vi "ImportExperiment.vi"(8 "error in (no error)":errorcluster, 10 "Tuple":T1={"mouse_id"=1217.0, "exp_date"="", "operator"="Manolis", "mass"=0.0, "anesthesia"="fentanyl", "directory"="", "dyes"="OGB", "exp_notes"="", "setup"="2P1", "archive"="", "process"="yes"}, 11 "Database in":refnum<class "Database.lvclass">) -> (0 "error out":errorcluster, 3 "Database out":refnum<class "Database.lvclass">)   [LabVIEW 2014, in "Database.lvclass"]
uses:
  Database.lvclass
  Database.lvclass/Database.ctl
  <vilib>/addons/database/NI_Database_API.lvlib
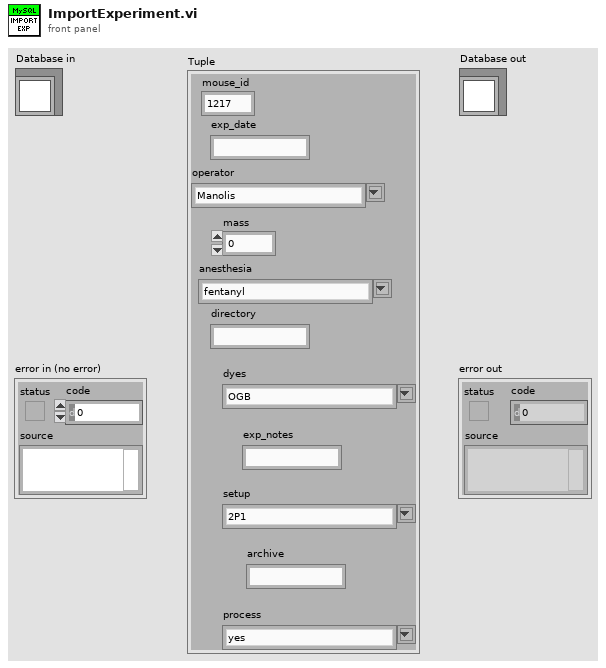
[diagram p1: front panel]
types:
  T1 = cluster{"mouse_id":dbl, "exp_date":string, "operator":string, "mass":dbl, "anesthesia":string, "directory":string, "dyes":string, "exp_notes":string, "setup":string, "archive":string, "process":string}
  T2 = typedef "NI_Database_API.lvlib/Conn ObjectReference.ctl" = refnum<k1>
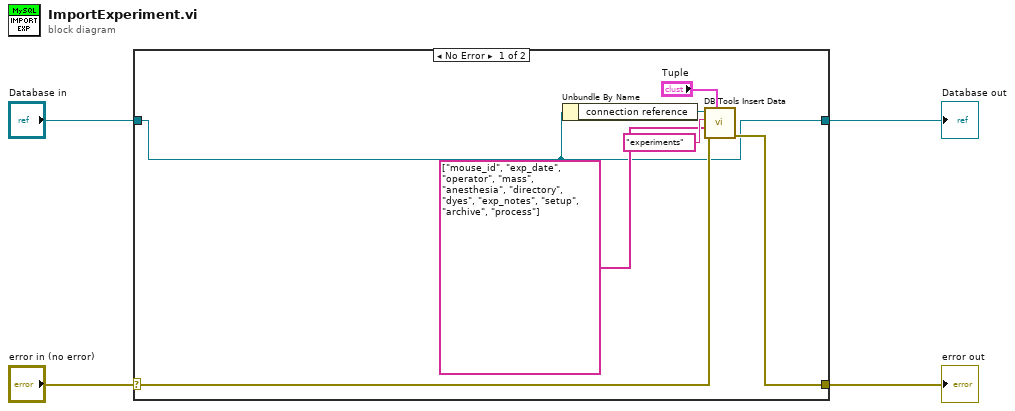
[diagram p0: block diagram]
diagram:
  n1 = case shown="No Error" "error in (no error)" {
    selector: "error in (no error)" -> [w7 w13]
    tunnel: [w6 w13] -> w3
    tunnel: [w5 w12] -> w1
    tunnel: "Database in" -> [w5 w12]
    frame No Error {
      n2 = Unbundle By Name(w5) -> ("connection reference"=w10:T2)
      n3 = call <vilib>:"DB Tools Insert Data.vi"("data"="Tuple", "error in (no error)"=w7, "columns"=string[] ["mouse_id", "exp_date", "operator", "mass", "anesthesia", "directory", "dyes", "exp_notes", "setup", "archive", "process"], "table"="experiments", "connection reference"=w10) -> ("error out"=w6:errorcluster)  [unwired: 5 in, 1 out]
    }
    frame Error {
    }
  }
  "error out" <- w3
  "Database out" <- w1
